vi "FVI_Manette_Swerve_Process.vi"(0 "Axe L X":dbl, 1 "Ltrigger":dbl, 2 "Rtrigger":dbl, 5 "Axe L Y":dbl, 7 "Axe R X":dbl, 9 "Axe R Y":dbl, 11 "POV":dbl, 12 "type mouvement":T2=enum."1 vitesse") -> (4 "SwerveDrive":T3)   [LabVIEW 2018]
uses:
  SwerveDrive.ctl
  Drivetype.ctl
  Direction 4 roues.ctl
  MyGlobal.vi
panel:
  in  "true or false face":bool=TRUE
  out "Correction angle":dbl
  out "4 roues":T1 {"ARD"."Vitesse" scale=-1.0..1.0; "ARD"."Angle" scale=-180.0..180.0; "ARG"."Vitesse" scale=-1.0..1.0; "ARG"."Angle" scale=-180.0..180.0; "AVD"."Vitesse" scale=-1.0..1.0; "AVD"."Angle" scale=-180.0..180.0; "AVG"."Vitesse" scale=-1.0..1.0; "AVG"."Angle" scale=-180.0..180.0}
  out "error out":errorcluster
  in  "error in (no error)":errorcluster
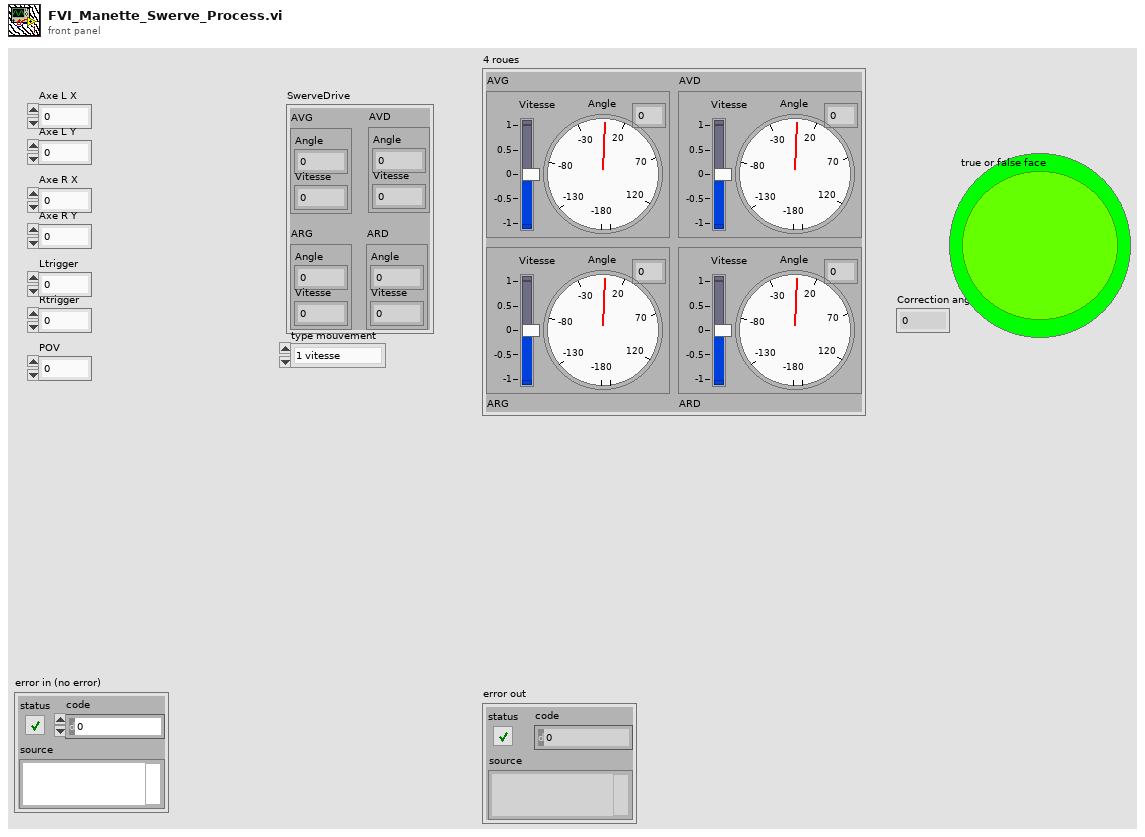
[diagram p1: front panel]
types:
  T1 = typedef "Direction 4 roues.ctl" = cluster{"AVG":cluster{"Angle":dbl, "Vitesse":dbl}, "AVD":cluster{"Angle":dbl, "Vitesse":dbl}, "ARG":cluster{"Angle":dbl, "Vitesse":dbl}, "ARD":cluster{"Angle":dbl, "Vitesse":dbl}}
  T2 = typedef "Drivetype.ctl" = enum16{"4 vitesse", "1 vitesse"}
  T3 = typedef "SwerveDrive.ctl" = cluster{"AVD":cluster{"Angle":dbl, "Vitesse":dbl}, "AVG":cluster{"Angle":dbl, "Vitesse":dbl}, "ARG":cluster{"Angle":dbl, "Vitesse":dbl}, "ARD":cluster{"Angle":dbl, "Vitesse":dbl}}
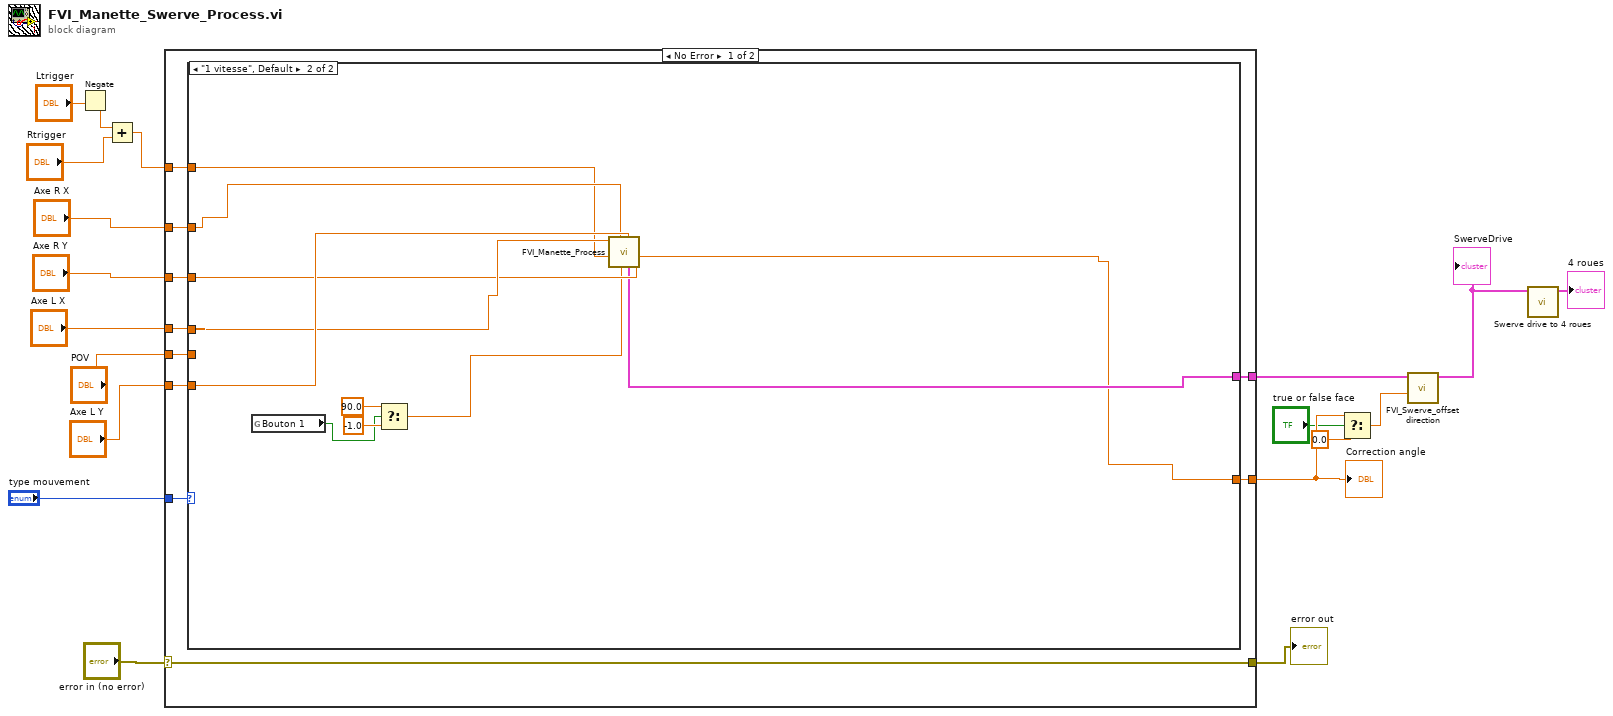
[diagram p0: block diagram]
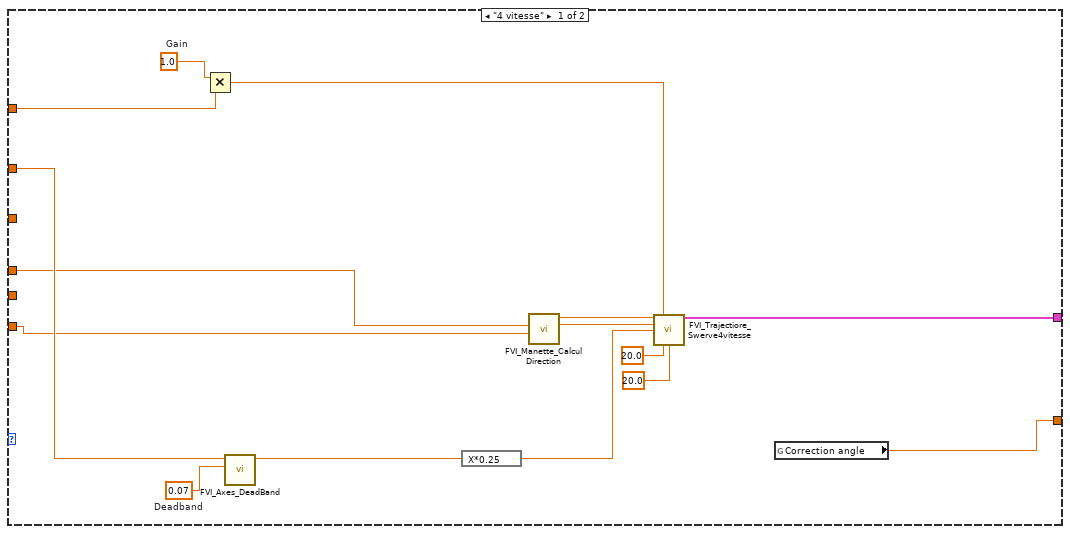
[diagram p2: hidden frame]
diagram:
  n1 = Negate(x="Ltrigger") -> (-x=w13:dbl)
  n2 = Add(x=w13, y="Rtrigger") -> (x+y=w11:dbl)
  n3 = case shown="No Error" "error in (no error)" {
    selector: "error in (no error)" -> [w29 w56]
    tunnel: "Axe L X" -> [w28 _]
    tunnel: "Axe L Y" -> [w27 _]
    tunnel: [w29 w56] -> w17
    tunnel: w11 -> [w24 _]
    tunnel: "POV" -> [w22 _]
    tunnel: "Axe R X" -> [w26 _]
    tunnel: "Axe R Y" -> [w21 _]
    tunnel: [w25 _] -> w6
    tunnel: "type mouvement" -> [w23 _]
    tunnel: [w20 _] -> w4
    frame No Error {
      n4 = case shown="\"1 vitesse\", Default" w23 {
        tunnel: w28 -> [w32 w53]
        tunnel: w27 -> [w31 w55]
        tunnel: w26 -> [w44 w54]
        tunnel: [w43 w50] -> w25
        tunnel: w24 -> [w37 w51]
        tunnel: w22 -> [_ _]
        tunnel: w21 -> [_ w52]
        tunnel: [w30 w49] -> w20
        frame "4 vitesse" {
          w42 = 0.07  # Deadband
          w34 = 1.0  # Gain
          n5 = Multiply(x=w34, y=w37) -> (x*y=w33:dbl)
          n6 = call "FVI_Axes_DeadBand.vi"("deadband Value"=w42, "X axis in"=w44) -> ("X axis out"=w40:dbl)  [unwired: 8 in, 1 out]
          n7 = expression code="X*0.25"(w40) -> (w35:dbl)
          n8 = call "FVI_Manette_Calcul Direction.vi"("Axe L Y"=w31, "Axe L X"=w32) -> ("Y"=w39:dbl, "X"=w38:dbl)  [unwired: 6 in, 2 out]
          n9 = call "FVI_Trajectiore_Swerve4vitesse.vi"("Vx"=w38, "Gain"=w33, "Vy"=w39, "Omega"=w35, "Longueur"=20.0 ("Distance"), "Largeur"=20.0) -> ("SwerveDrive"=w43:T3)  [unwired: 9 in]
          n10 = global read "MyGlobal.vi" "Correction angle"() -> (w30:dbl)
        }
        frame "1 vitesse", Default {
          n11 = global read "MyGlobal.vi" "Bouton 1"() -> (w46:bool)
          n12 = Select(t=90.0, s=w46, f=-1.0) -> (s? t:f=w45:dbl)
          n13 = call "FVI_Manette_Process.vi"("Axe R Y"=w52, "Axe L Y"=w55, "POV"=w45, "Axe R X"=w54, "Rtrigger"=w51, "Axe L X"=w53) -> ("Correction angle"=w49:dbl, "SwerveDrive"=w50:T3)  [unwired: 4 in]
        }
      }
    }
    frame Error {
    }
  }
  "error out" <- w17
  "Correction angle" <- w4
  n14 = Select(t=w4, s="true or false face", f=0.0) -> (s? t:f=w1:dbl)
  n15 = call "FVI_Swerve_offset direction.vi"("Correction angle"=w1, "SwerveDrive in"=w6) -> ("SwerveDrive out"=w5:T3)  [unwired: 9 in]
  "SwerveDrive" <- w5
  n16 = call "Swerve drive to 4 roues.vi"("SwerveDrive"=w5) -> ("4 roues"=→"4 roues":T1)  [unwired: 10 in]
